vi "SGDA-Start.vi"(4 "error in (no error)":errorcluster, 5 "wait for DAQ? (F)":bool) -> (0 "error out":errorcluster)   [LabVIEW 2020]
doc: "Sends <B>Start</B> notifier to DAQ thread to begin measurement."
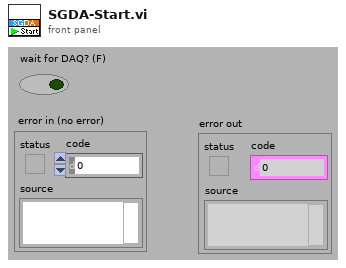
[diagram p1: front panel]
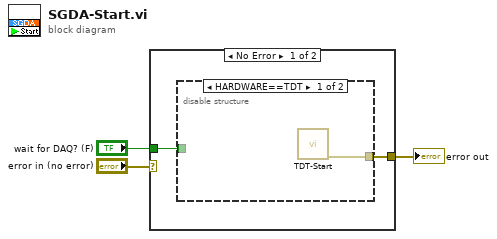
[diagram p0: block diagram]
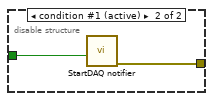
[diagram p2: hidden frame]
diagram:
  n1 = case shown="No Error" "error in (no error)" {
    selector: "error in (no error)" -> [_ w9]
    tunnel: "wait for DAQ? (F)" -> [w5 _]
    tunnel: [w4 w9] -> w1
    frame No Error {
      n2 = disable-structure shown="HARDWARE==TDT" {
        disable-tunnel: w5 -> [_ w8]
        disable-tunnel: [w6 w7] -> w4
        frame condition #0 {
          n3 = call "TDT-Start.vi"() -> ("error out"=w6:errorcluster)  [unwired: 7 in]
        }
        frame condition #1 (active) {
          n4 = call "StartDAQ notifier.vi"("wait for DAQ? (F)"=w8) -> ("error out"=w7:errorcluster)  [unwired: 6 in]
        }
      }
    }
    frame Error {
    }
  }
  "error out" <- w1
